vi "auto_regex.vi"(8 "error in (no error)":errorcluster, 10 "Regex":string[][](array[string]), 11 "SN":string) -> (0 "error out":errorcluster, 1 "Device Type out":T1, 2 "SN ok?":bool, 3 "SN out":string)   [LabVIEW 2024]
uses:
  controls/SN_device_type_out.ctl
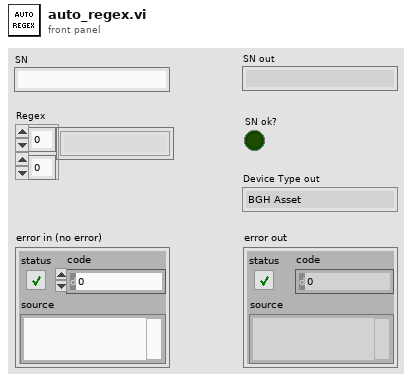
[diagram p1: front panel]
types:
  T1 = typedef "SN_device_type_out.ctl" = enum16{"BGH Asset", "BGH Product", "SAMSUNG Product", "GENERIC Product", "No Product", "_"}
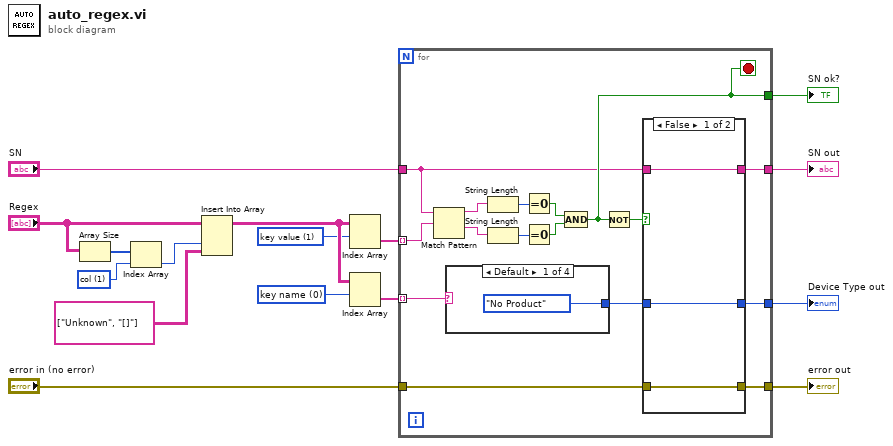
[diagram p0: block diagram]
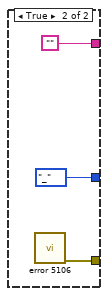
[diagram p2: hidden frame]
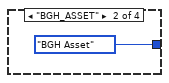
[diagram p3: hidden frame]
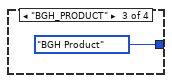
[diagram p4: hidden frame]
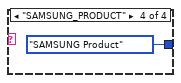
[diagram p5: hidden frame]
diagram:
  w5 = 1 items=["row", "col"]
  w11 = 1 items=["key name", "key value"]
  w12 = 0 items=["key name", "key value"]
  n1 = Array Size(array="Regex") -> (size(s)=w10:i32[])
  n2 = Index Array(array=w10, index=w5) -> (element=w9:i32)
  n3 = Insert Into Array "Insert Into Array"(array="Regex", index (col)=w9, new element=string[][] [["Unknown"], ["[]"]]) -> (w13:string[][])  [unwired: 1 in]
  n4 = Index Array(array=w13, index (row)=w11) -> (element=w15:string[])  [unwired: 1 in]
  n5 = Index Array(array=w13, index (row)=w12) -> (element=w16:string[])  [unwired: 1 in]
  n6 = for {
    tunnel: w16 -> [w32] mode=indexing
    tunnel: w15 -> [w25] mode=indexing
    tunnel: "SN" -> [w18]
    tunnel: [w22] -> w6
    tunnel: [w24] -> w7
    tunnel: [w20] -> w3
    tunnel: "error in (no error)" -> [w19]
    tunnel: [w17] -> w1
    stop <- w24 stop-if-true
    n7 = Match Pattern(string=w18, regular expression=w25) -> (before substring=w26:string, after substring=w27:string)  [unwired: 1 in, 2 out]
    n8 = case shown="Default" w32 {
      tunnel: [SN_device_type_out."No Product" ("Device Type out") SN_device_type_out."BGH Asset" ("Device Type out") SN_device_type_out."BGH Product" ("Device Type out") SN_device_type_out."SAMSUNG Product" ("Device Type out")] -> w23
      frame Default {
      }
      frame "BGH_ASSET" {
      }
      frame "BGH_PRODUCT" {
      }
      frame "SAMSUNG_PRODUCT" {
      }
    }
    n9 = String Length(string=w26) -> (length=w28:i32)
    n10 = String Length(string=w27) -> (length=w29:i32)
    n11 = Equal To 0?(x=w28) -> (x = 0?=w31:bool)
    n12 = Equal To 0?(x=w29) -> (x = 0?=w30:bool)
    n13 = Compound Arithmetic op=AND(w31, w30) -> (w24:bool)
    n14 = Not(x=w24) -> (.not. x?=w21:bool)
    n15 = case shown="False" w21 {
      tunnel: [w35 SN_device_type_out."_" ("t")] -> w22
      tunnel: w23 -> [w35 _]
      tunnel: [w34 w37] -> w20
      tunnel: w19 -> [w34 _]
      tunnel: w18 -> [w33 _]
      tunnel: [w33 ""] -> w17
      frame False {
      }
      frame True {
        n16 = call "error 5106.vi"() -> ("error out"=w37:errorcluster)  [unwired: 11 in]
      }
    }
  }
  "SN ok?" <- w7
  "Device Type out" <- w6
  "error out" <- w3
  "SN out" <- w1
